vi "RemoveChildFromNode.vi"(8 "error in":errorcluster, 10 "removed child":T1, 11 "CEF_serializable node folder in":refnum<class "CEF_serializable node folder.lvclass">) -> (0 "error out":errorcluster, 3 "CEF_serializable node folder out":refnum<class "CEF_serializable node folder.lvclass">)   [LabVIEW 2023, in "CEF_serializable node folder.lvclass"]
doc: "Copyright 2017 National Instruments Corporation\n\nLicensed under the Apache License, Version 2.0 (the \"License\"); you may not use this file except in compliance with the License. You may obtain a copy of the License at http://www.apache.org/licenses/LICENSE-2.0\nUnless required by applicable law or agreed to in writing, software distributed under the License is distributed on an \"AS IS\" BASIS, WITHOUT WARRANTIES OR CONDITIONS OF ANY KIND, either express or implied. See the License for the specific language governing permissions and limitations under the License."
uses:
  CEF_serializable node folder.lvclass
  <vilib>/NI/Configuration Framework/Node/NodeRef.ctl
  <vilib>/NI/Configuration Framework/Node/NISE_CEF_Node.lvclass
  <vilib>/NI/Configuration Framework/Node/NISE_CEF_Node.lvclass/NISE_CEF_Node.ctl
  <vilib>/NI/Configuration Framework/Node/ReadParent.vi
  serializable node/NISE_CEF_serializable node.lvclass
  CEF_serializable node folder.lvclass/CEF_serializable node folder.ctl
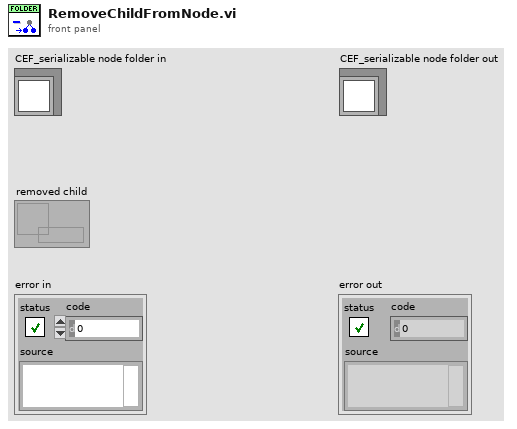
[diagram p1: front panel]
types:
  T1 = typedef "NISE_CEF_Node.lvclass/NodeRef.ctl" = refnum<data-value>
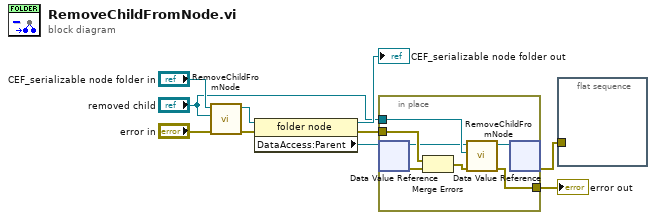
[diagram p0: block diagram]
diagram:
  n1 = call-parent "RemoveChildFromNode.vi"("error in"="error in", "removed child"="removed child", "NISE_CEF_Node in"="CEF_serializable node folder in") -> ("error out"=w10:errorcluster, "NISE_CEF_Node out"=w7:refnum<class "CEF_serializable node folder.lvclass">)  [unwired: 7 in]
  n2 = property class="folder node"(reference=w7, error in=w10) -> (reference out=→"CEF_serializable node folder out":refnum<class "CEF_serializable node folder.lvclass">, error out=w5:errorcluster, "DataAccess:Parent"=w2:T1)
  n3 = in-place {
    in-place-border: w5 -> [w17]
    in-place-border: [w16] -> w4
    in-place-border: "removed child" -> [w15]
    n4 = in-place-dvr #1(w2) -> (w14:refnum<class "NISE_CEF_Node.lvclass">, w11:errorcluster)
    n5 = Merge Errors(w17, w11) -> (w12:errorcluster)
    n6 = call-dynamic "RemoveChildFromNode.vi"("error in"=w12, "removed child"=w15, "NISE_CEF_Node in"=w14) -> ("error out"=w16:errorcluster, "NISE_CEF_Node out"=w13:refnum<class "NISE_CEF_Node.lvclass">)  [unwired: 7 in]
    n7 = in-place-dvr #1(w13) -> (w1:errorcluster)  [unwired: 1 out]
  }
  "error out" <- w4
  n8 = flat-sequence {
    tunnel: w1 -> [_]
    frame #0 {
    }
  }
